vi "通用虚拟串口配置范例.vi"() -> ()   [LabVIEW 2013]
uses:
  <vilib>/Instr/_visa.llb/VISA Find Search Mode.ctl
  <vilib>/Instr/_visa.llb/VISA Set IO Buffer Mask.ctl
  <vilib>/Instr/_visa.llb/VISA Configure Serial Port (Instr).vi
panel:
  out "BUSY":bool
  in  "报警值":dbl format="%#_13g"
  in  "数量级单位":cluster{"数量级":u16, "单位":u16}={"数量级"=3, "单位"=1} {"单位" items=["Gy/h"=1, "Sv/h"=2, "CPS"=3, "Bq/cm2"=4, "Sv"=5]; "数量级" items=["μ(微)"=2, "m(毫)"=3, "--(无前缀)"=4, "k(千)"=5]}
  out "CRC？":bool
  in  "(其他)等待字节数(4096)":u32=1700
  in  "(实时)等待字节数(4096)":u32=17
  out "读取时间s":dbl
  out "主探测器":T1={"测量值"=0.0, "数量级"=2, "单位"=1, "单位字符串"=""} {"单位" items=["Gy/h"=1, "Sv/h"=2, "CPS"=3, "Bq/cm2"=4, "Sv"=5]; "数量级" items=["n"=1, "μ"=2, "m"=3, " "=4, "k"=5]; "测量值" format="%.2g"}
  in  "报警方式":T2={"声音.1"=TRUE, "闪灯.2"=TRUE, "寻源.8"=TRUE, "震动.4"=TRUE}
  out "输出数组":string[](array[string])
  in  "停止按钮":bool
  out "返回数":u32
  in  "VISA资源名称":refnum<visa-resource-name>="COM10"
  out "错误输出":errorcluster
  out "查找列表":string[](array[string])
  out "读取缓冲区":string
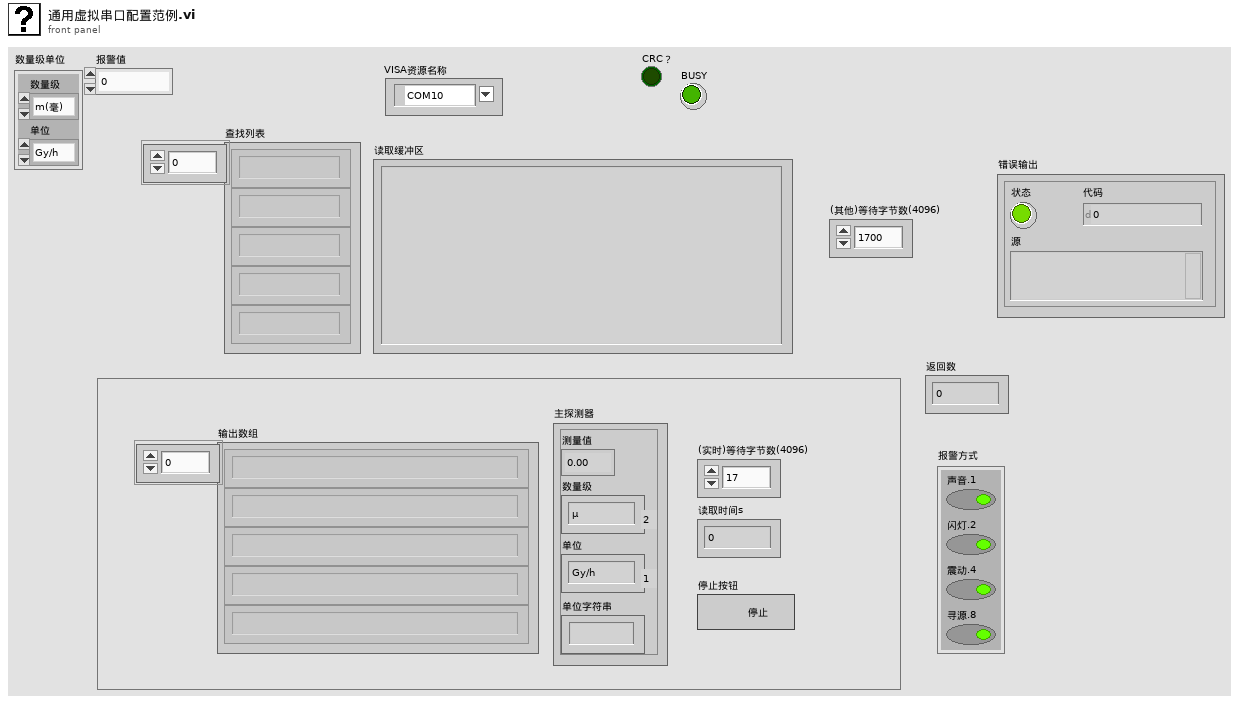
[diagram p1: front panel]
types:
  T1 = cluster{"测量值":dbl, "数量级":u16, "单位":u16, "单位字符串":string}
  T2 = cluster{"声音.1":bool, "闪灯.2":bool, "寻源.8":bool, "震动.4":bool}
  T3 = typedef "VISA Find Search Mode.ctl" = u32
  T4 = typedef "VISA Set IO Buffer Mask.ctl" = u16
  T5 = enum16{"中间数据(Min<x<Max)", "最新数据(x>Max)", "最旧数据(x<Min)"}
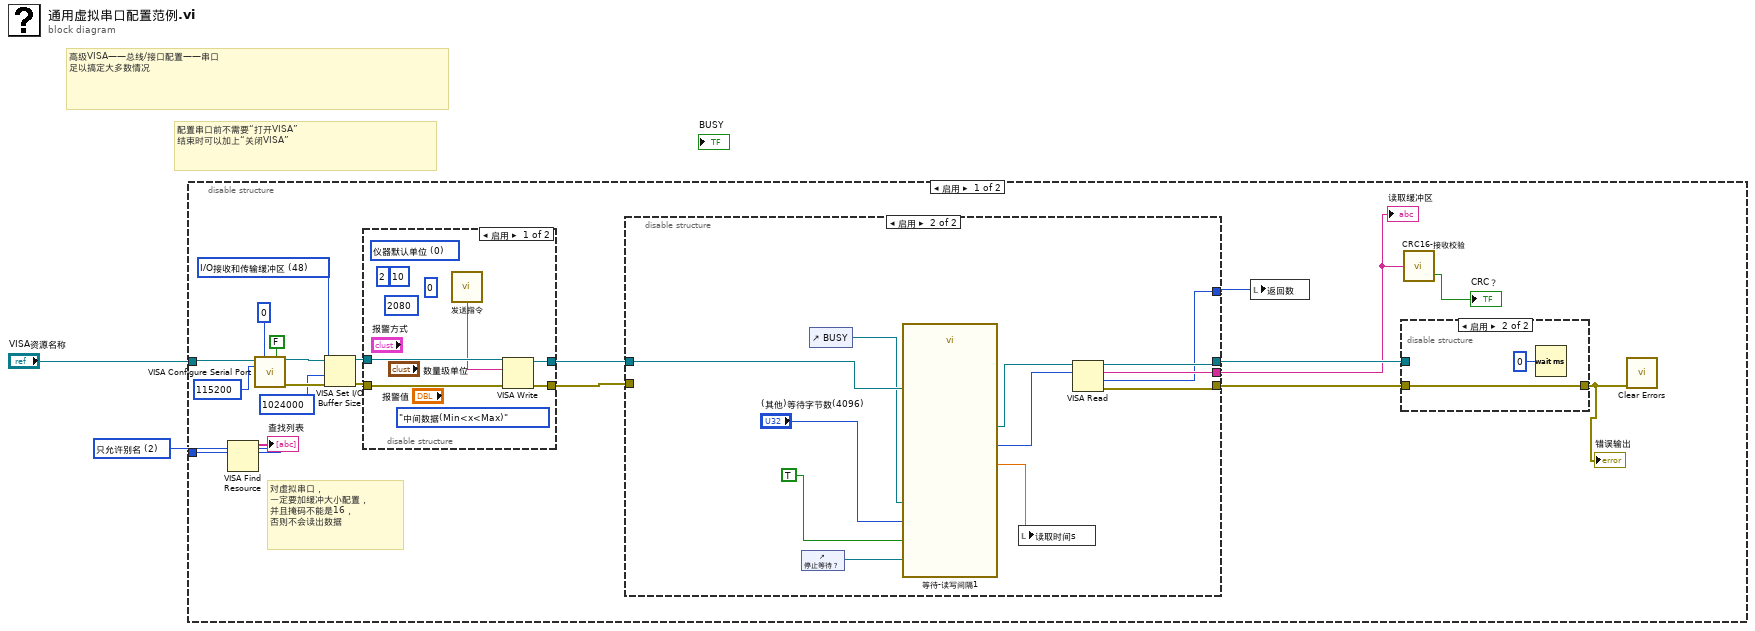
[diagram p0: block diagram]
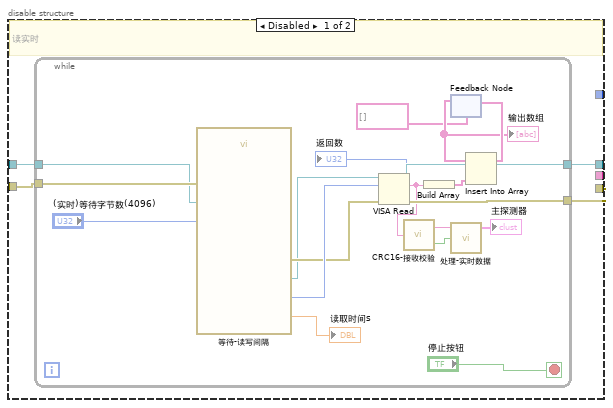
[diagram p2: hidden frame]
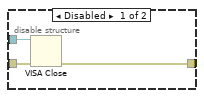
[diagram p3: hidden frame]
diagram:
  w2 = T3 2 items=["仅允许规范名称"=0, "只允许别名"=2, "包含匹配别名"=3, "包含所有别名"=4] ("Search Mode")
  # "高级VISA——总线/接口配置——串口\n足以搞定大多数情况"
  # "配置串口前不需要“打开VISA”\n结束时可以加上“关闭VISA”"
  n1 = disable-structure shown="启用" {
    disable-tunnel: w2 -> [w22 _]
    disable-tunnel: "VISA资源名称" -> [w19 _]
    frame Enabled {
      w7 = T4 48 items=["I/O接收缓冲区"=16, "I/O传输缓冲区"=32, "I/O接收和传输缓冲区"=48] ("Mask")
      # "对虚拟串口，\n一定要加缓冲大小配置，\n并且掩码不能是16，\n否则不会读出数据"
      n2 = VISA Find Resource(10:w22) -> (3:→"查找列表":string[])  [unwired: 2 in, 2 out]
      n3 = call-poly "VISA Configure Serial Port"("VISA resource name"=w19, "timeout (10sec)"=u32 0, "Enable Termination\nChar (T)"=FALSE ("Enable Termination\nChar (T)"), "baud rate (9600)"=u32 115200) -> ("VISA resource name out"=w18:refnum<visa-resource-name>, "error out"=w16:errorcluster)  [unwired: 10 in]
      n4 = VISA Set I/O Buffer Size(VISA resource name=w18, mask (16)=w7, size (4096)=u32 1024000 ("大小(4096)"), error in (no error)=w16) -> (VISA resource name out=w14:refnum<visa-resource-name>, error out=w13:errorcluster)
      n5 = disable-structure shown="启用" {
        disable-tunnel: [w67 w69] -> w20
        disable-tunnel: [w66 w68] -> w9
        disable-tunnel: w14 -> [w65 w69]
        disable-tunnel: w13 -> [w64 w68]
        frame Enabled {
          (unwired) u16 0 ("Max")
          (unwired) u8 2 ("报警等级")
          (unwired) u16 10 ("采样时间(0~999s)")
          (unwired) u16 0 items=["仪器默认单位", "Gy/h", "Sv/h", "CPS", "Bq/cm2", "Sv"] ("单位选择")
          (unwired) u16 2080 ("Max")
          (unwired) T5."中间数据(Min<x<Max)" ("读取模式")
          n6 = call-poly "发送指令.vi"() -> ("读MAC与型号-8w"=w63:string)  [unwired: 3 in]
          n7 = VISA Write(VISA resource name=w65, write buffer=w63, error in (no error)=w64) -> (VISA resource name out=w67:refnum<visa-resource-name>, error out=w66:errorcluster)  [unwired: 1 out]
        }
        frame Disabled {
        }
      }
      n8 = disable-structure shown="启用" {
        disable-tunnel: w9 -> [w26 _]
        disable-tunnel: w20 -> [w25 w55]
        disable-tunnel: [w24 w53] -> w10
        disable-tunnel: [w23 w52] -> w11
        disable-tunnel: [_ w54] -> w6
        disable-tunnel: [_ w49] -> w5
        frame Disabled {
          # "读实时"
          n9 = while {
            tunnel: w26 -> [w45]
            tunnel: w25 -> [w44]
            tunnel: [w40] -> w24
            tunnel: [w39] -> w23
            stop <- "停止按钮" stop-if-true
            n10 = call "等待-读写间隔.vi"("error in"=w45, "等待字节数(4096)"="(实时)等待字节数(4096)", "VISA资源名i"=w44) -> ("error out"=w42:errorcluster, "读取时间s"=→"读取时间s":dbl, "读取字节数"=w43:u32, "VISA资源名o"=w41:refnum<visa-resource-name>)  [unwired: 4 in, 1 out]
            n11 = VISA Read(VISA resource name=w41, byte count=w43, error in (no error)=w42) -> (VISA resource name out=w40:refnum<visa-resource-name>, read buffer=w32:string, return count=→"返回数":u32, error out=w39:errorcluster)
            n12 = call "CRC16-接收校验.vi"("读取缓冲区"=w32) -> ("净数据"=w30:string, "CRC？"=w31:bool)
            n13 = Build Array(w32) -> (w37:string[])
            n14 = feedback #1(string[] []) -> (w35:string[])
            "输出数组" <- w35
            n15 = call "处理-实时数据.vi"("CRC？"=w31, "净数据"=w30) -> ("主探测器"=→"主探测器":T1)  [unwired: 1 in, 2 out]
            n16 = Insert Into Array(array=w35, new element=w37) -> (w36:string[])  [unwired: 1 in]
            n17 = feedback-in #1(w36) -> ()
          }
        }
        frame Enabled {
          n18 = control-ref of="停止等待？"() -> (w47:refnum<vi>)
          n19 = control-ref of="BUSY"() -> (w48:refnum<vi>)
          n20 = call "等待-读写间隔1.vi"("BUSY引用"=w48, "强制停止？引用"=w47, "忙时等待？"=TRUE, "等待字节数(500k)"="(其他)等待字节数(4096)", "VISA资源名i"=w55) -> ("读取时间s"=w50:dbl, "读取字节数"=w57:u32, "VISA资源名o"=w56:refnum<visa-resource-name>)  [unwired: 3 in, 1 out]
          n21 = local write "读取时间s"(w50) -> ()
          n22 = VISA Read(VISA resource name=w56, byte count=w57) -> (VISA resource name out=w53:refnum<visa-resource-name>, read buffer=w54:string, return count=w49:u32, error out=w52:errorcluster)  [unwired: 1 in]
        }
      }
      "读取缓冲区" <- w6
      n23 = local write "返回数"(w5) -> ()
      n24 = disable-structure shown="启用" {
        disable-tunnel: w11 -> [w60 w62]
        disable-tunnel: w10 -> [w59 _]
        disable-tunnel: [w58 w62] -> w8
        frame Disabled {
          n25 = VISA Close(VISA resource name=w59, error in (no error)=w60) -> (error out=w58:errorcluster)
        }
        frame Enabled {
          n26 = Wait (ms)(milliseconds to wait=u32 0 ("等待时间（毫秒）")) -> ()  [unwired: 1 out]
        }
      }
      "错误输出" <- w8
      n27 = call "CRC16-接收校验.vi"("读取缓冲区"=w6) -> ("CRC？"=→"CRC？":bool)  [unwired: 1 out]
      n28 = call <vilib>:"Clear Errors.vi"("error in (no error)"=w8) -> ()  [unwired: 6 in, 1 out]
    }
    frame Disabled {
    }
  }
